vi "create-child.vi"(5 "max (10)":dbl=10.0, 7 "min (0)":dbl, 8 "error in":errorcluster, 9 "physical channel":string, 10 "name":string, 11 "channel-child in":refnum<class "channel-child.lvclass">) -> (0 "error out":errorcluster, 3 "channel-child out":refnum<class "channel-child.lvclass">)   [LabVIEW 2020, in "channel-child.lvclass"]
uses:
  channel-child/channel-child.lvclass
  C:/code/sandbox/serialization/test-channel/test-channel.lvclass
  channel-child/channel-child.lvclass/channel-child.ctl
  test-channel/test-channel.lvclass
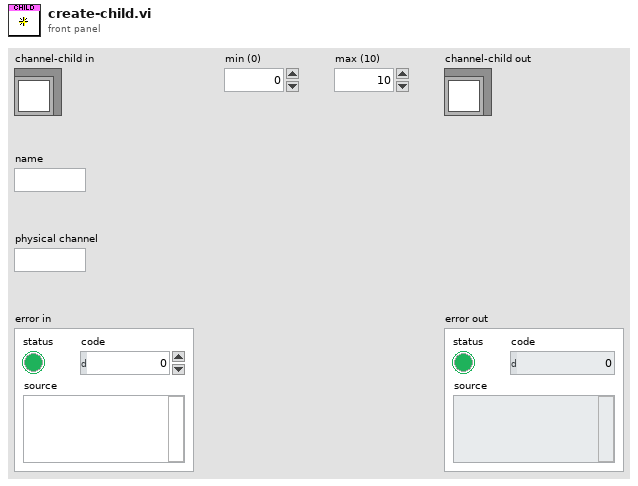
[diagram p1: front panel]
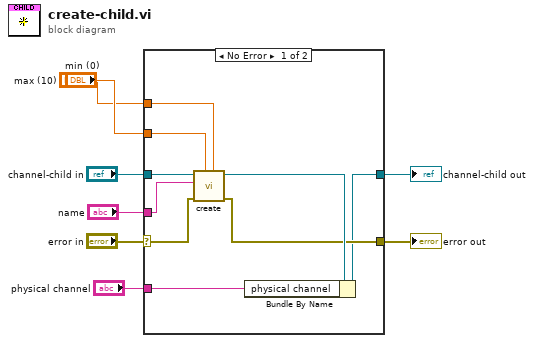
[diagram p0: block diagram]
diagram:
  n1 = case shown="No Error" "error in" {
    selector: "error in" -> [w15 w19]
    tunnel: [w14 w19] -> w7
    tunnel: [w10 w18] -> w5
    tunnel: "channel-child in" -> [w16 w18]
    tunnel: "min (0)" -> [w13 _]
    tunnel: "max (10)" -> [w12 _]
    tunnel: "name" -> [w11 _]
    tunnel: "physical channel" -> [w9 _]
    frame No Error {
      n2 = call "create.vi"("max (10)"=w12, "min (0)"=w13, "error in"=w15, "name"=w11, "test-channel in"=w16) -> ("error out"=w14:errorcluster, "test-channel out"=w17:refnum<class "channel-child.lvclass">)  [unwired: 5 in]
      n3 = Bundle By Name(cluster=w17, "physical channel"=w9) -> (w10:refnum<class "channel-child.lvclass">)
    }
    frame Error {
    }
  }
  "error out" <- w7
  "channel-child out" <- w5
